vi "DOE Kitchen Data MW100 Compile.vi"(7 "TC Coefficients":T1, 8 "Error In":errorcluster, 10 "Data Input":dbl[](array[numeric])) -> (0 "Error Out":errorcluster, 3 "Kitchen Cluster":T2)   [LabVIEW 2016]
uses:
  Type Definitions/DOE Kitchen Control.ctl
  Utility/Type Definitions/UTILITY TC Coefficients.ctl
  Utility/Type Definitions/UTILITY TC Coefficients Selector.ctl
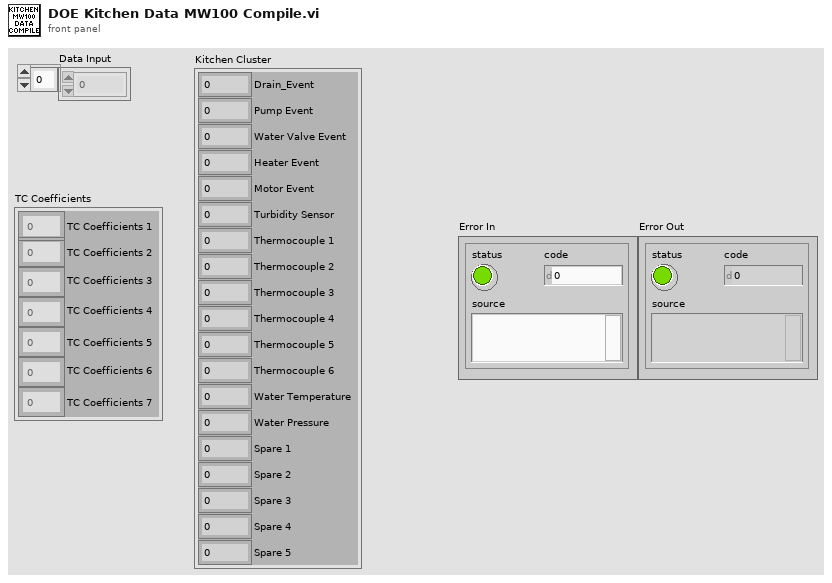
[diagram p1: front panel]
types:
  T1 = typedef "UTILITY TC Coefficients.ctl" = cluster{"TC Coefficients 1":dbl[], "TC Coefficients 2":dbl[], "TC Coefficients 3":dbl[], "TC Coefficients 4":dbl[], "TC Coefficients 5":dbl[], "TC Coefficients 6":dbl[], "TC Coefficients 7":dbl[]}
  T2 = typedef "DOE Kitchen Control.ctl" = cluster{"Drain_Event":i16, "Pump Event":i16, "Water Valve Event":i16, "Heater Event":i16, "Motor Event":i16, "Turbidity Sensor":dbl, "Thermocouple 1":dbl, "Thermocouple 2":dbl, "Thermocouple 3":dbl, "Thermocouple 4":dbl, "Thermocouple 5":dbl, "Thermocouple 6":dbl, "Water Temperature":dbl, "Water Pressure":dbl, "Spare 1":dbl, "Spare 2":dbl, "Spare 3":dbl, "Spare 4":dbl, "Spare 5":dbl}
  T3 = typedef "UTILITY TC Coefficients Selector.ctl" = enum16{"TC1", "TC2", "TC3", "TC4", "TC5", "TC6", "TC7"}
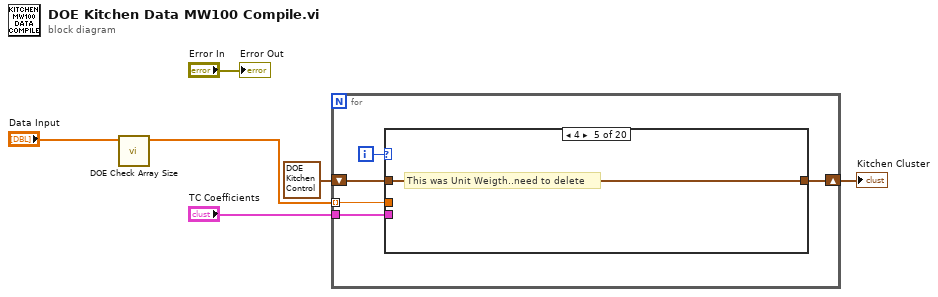
[diagram p0: block diagram]
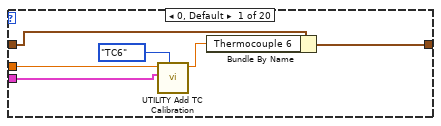
[diagram p2: hidden frame]
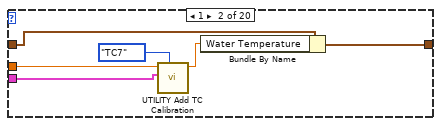
[diagram p3: hidden frame]
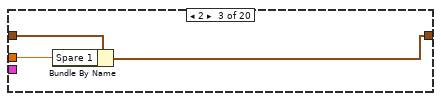
[diagram p4: hidden frame]
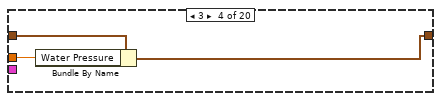
[diagram p5: hidden frame]
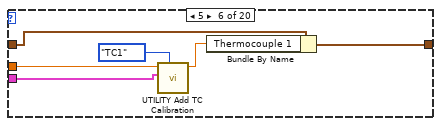
[diagram p6: hidden frame]
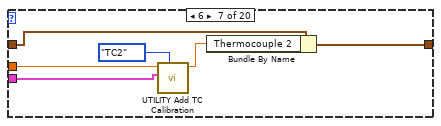
[diagram p7: hidden frame]
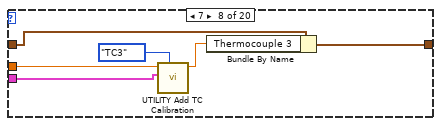
[diagram p8: hidden frame]
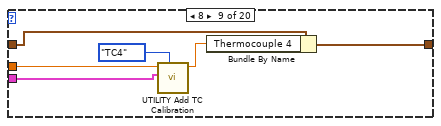
[diagram p9: hidden frame]
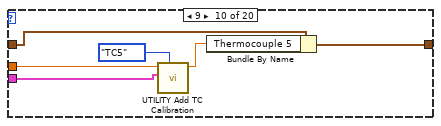
[diagram p10: hidden frame]
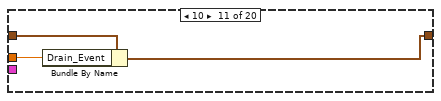
[diagram p11: hidden frame]
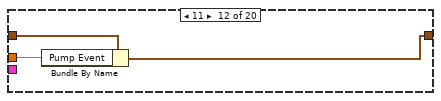
[diagram p12: hidden frame]
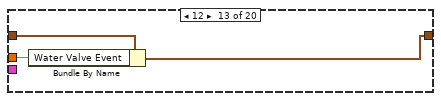
[diagram p13: hidden frame]
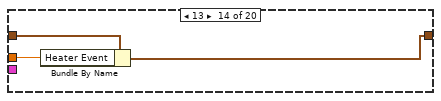
[diagram p14: hidden frame]
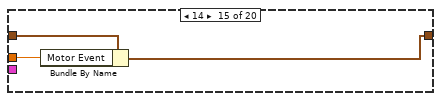
[diagram p15: hidden frame]
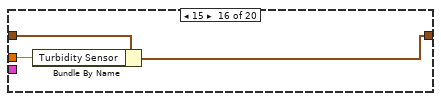
[diagram p16: hidden frame]
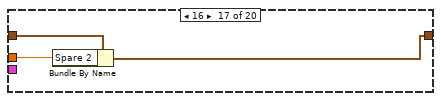
[diagram p17: hidden frame]
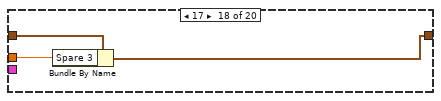
[diagram p18: hidden frame]
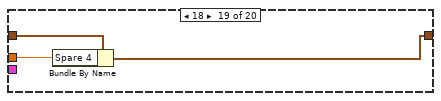
[diagram p19: hidden frame]
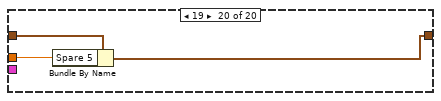
[diagram p20: hidden frame]
diagram:
  n1 = call "DOE Check Array Size.vi"("Data List"="Data Input") -> ("Output Array"=w1:dbl[])  [unwired: 9 in, 1 out]
  n2 = for {
    tunnel: w1 -> [w8] mode=indexing
    shift-right: [w9] -> w5
    shift-left: T2 {"Drain_Event"=0, "Pump Event"=0, "Water Valve Event"=0, "Heater Event"=0, "Motor Event"=0, "Turbidity Sensor"=0.0, "Thermocouple 1"=0.0, "Thermocouple 2"=0.0, "Thermocouple 3"=0.0, "Thermocouple 4"=0.0, "Thermocouple 5"=0.0, "Thermocouple 6"=0.0, "Water Temperature"=0.0, "Water Pressure"=0.0, "Spare 1"=0.0, "Spare 2"=0.0, "Spare 3"=0.0, "Spare 4"=0.0, "Spare 5"=0.0} -> [w10]
    tunnel: "TC Coefficients" -> [w7]
    i -> [w11]
    n3 = case shown="4" w11 {
      tunnel: w10 -> [w17 w23 w26 w29 w30 w36 w41 w48 w54 w60 w63 w66 w68 w72 w75 w78 w81 w84 w87 w90]
      tunnel: [w16 w22 w25 w28 w30 w35 w42 w47 w53 w59 w62 w65 w67 w71 w74 w77 w80 w83 w86 w89] -> w9
      tunnel: w8 -> [w14 w19 w24 w27 _ w32 w38 w44 w50 w56 w61 w64 w69 w70 w73 w76 w79 w82 w85 w88]
      tunnel: w7 -> [w15 w18 _ _ _ w31 w37 w43 w49 w55 _ _ _ _ _ _ _ _ _ _]
      frame 0, Default {
        n4 = call "UTILITY Add TC Calibration.vi"("Enum"=UTILITY_TC_Coefficients_Selector."TC6", "TC Coefficients"=w15, "Non Cal Temp"=w14) -> ("Calibrated Temp"=w13:dbl)  [unwired: 8 in]
        n5 = Bundle By Name(cluster=w17, "Thermocouple 6"=w13) -> (w16:T2)
      }
      frame 1 {
        n6 = call "UTILITY Add TC Calibration.vi"("Enum"=UTILITY_TC_Coefficients_Selector."TC7", "TC Coefficients"=w18, "Non Cal Temp"=w19) -> ("Calibrated Temp"=w20:dbl)  [unwired: 8 in]
        n7 = Bundle By Name(cluster=w23, "Water Temperature"=w20) -> (w22:T2)
      }
      frame 2 {
        n8 = Bundle By Name(cluster=w26, "Spare 1"=w24) -> (w25:T2)
      }
      frame 3 {
        n9 = Bundle By Name(cluster=w29, "Water Pressure"=w27) -> (w28:T2)
      }
      frame 4 {
        # "This was Unit Weigth..need to delete"
      }
      frame 5 {
        n10 = call "UTILITY Add TC Calibration.vi"("Enum"=UTILITY_TC_Coefficients_Selector."TC1", "TC Coefficients"=w31, "Non Cal Temp"=w32) -> ("Calibrated Temp"=w33:dbl)  [unwired: 8 in]
        n11 = Bundle By Name(cluster=w36, "Thermocouple 1"=w33) -> (w35:T2)
      }
      frame 6 {
        n12 = call "UTILITY Add TC Calibration.vi"("Enum"=UTILITY_TC_Coefficients_Selector."TC2", "TC Coefficients"=w37, "Non Cal Temp"=w38) -> ("Calibrated Temp"=w39:dbl)  [unwired: 8 in]
        n13 = Bundle By Name(cluster=w41, "Thermocouple 2"=w39) -> (w42:T2)
      }
      frame 7 {
        n14 = call "UTILITY Add TC Calibration.vi"("Enum"=UTILITY_TC_Coefficients_Selector."TC3", "TC Coefficients"=w43, "Non Cal Temp"=w44) -> ("Calibrated Temp"=w45:dbl)  [unwired: 8 in]
        n15 = Bundle By Name(cluster=w48, "Thermocouple 3"=w45) -> (w47:T2)
      }
      frame 8 {
        n16 = call "UTILITY Add TC Calibration.vi"("Enum"=UTILITY_TC_Coefficients_Selector."TC4", "TC Coefficients"=w49, "Non Cal Temp"=w50) -> ("Calibrated Temp"=w51:dbl)  [unwired: 8 in]
        n17 = Bundle By Name(cluster=w54, "Thermocouple 4"=w51) -> (w53:T2)
      }
      frame 9 {
        n18 = call "UTILITY Add TC Calibration.vi"("Enum"=UTILITY_TC_Coefficients_Selector."TC5", "TC Coefficients"=w55, "Non Cal Temp"=w56) -> ("Calibrated Temp"=w57:dbl)  [unwired: 8 in]
        n19 = Bundle By Name(cluster=w60, "Thermocouple 5"=w57) -> (w59:T2)
      }
      frame 10 {
        n20 = Bundle By Name(cluster=w63, "Drain_Event"=w61) -> (w62:T2)
      }
      frame 11 {
        n21 = Bundle By Name(cluster=w66, "Pump Event"=w64) -> (w65:T2)
      }
      frame 12 {
        n22 = Bundle By Name(cluster=w68, "Water Valve Event"=w69) -> (w67:T2)
      }
      frame 13 {
        n23 = Bundle By Name(cluster=w72, "Heater Event"=w70) -> (w71:T2)
      }
      frame 14 {
        n24 = Bundle By Name(cluster=w75, "Motor Event"=w73) -> (w74:T2)
      }
      frame 15 {
        n25 = Bundle By Name(cluster=w78, "Turbidity Sensor"=w76) -> (w77:T2)
      }
      frame 16 {
        n26 = Bundle By Name(cluster=w81, "Spare 2"=w79) -> (w80:T2)
      }
      frame 17 {
        n27 = Bundle By Name(cluster=w84, "Spare 3"=w82) -> (w83:T2)
      }
      frame 18 {
        n28 = Bundle By Name(cluster=w87, "Spare 4"=w85) -> (w86:T2)
      }
      frame 19 {
        n29 = Bundle By Name(cluster=w90, "Spare 5"=w88) -> (w89:T2)
      }
    }
  }
  "Kitchen Cluster" <- w5
  "Error Out" <- "Error In"
